vi "Find the boundary for Case Stucture.vi"(11 "Array 2":cluster{"Position":T1, "Bounds Rect":T2}[](array[cluster])) -> (0 "Height":i32, 1 "Width":i32, 2 "Top Min":i32, 3 "Left Min":i32)   [LabVIEW 2014]
uses:
  <vilib>/Utility/miscctls.llb/LVPositionTypeDef.ctl
  <vilib>/Utility/miscctls.llb/LVRectTypeDef.ctl
panel:
  out "Top Max":i32
  out "Left Max":i32
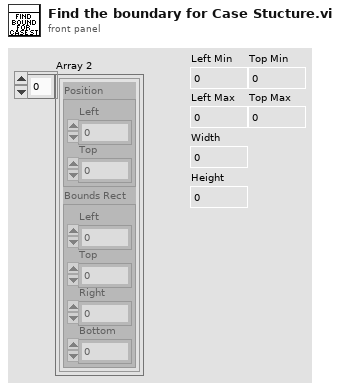
[diagram p1: front panel]
types:
  T1 = typedef "LVPositionTypeDef.ctl" = cluster{"Left":i32, "Top":i32}
  T2 = typedef "LVRectTypeDef.ctl" = cluster{"Left":i16, "Top":i16, "Right":i16, "Bottom":i16}
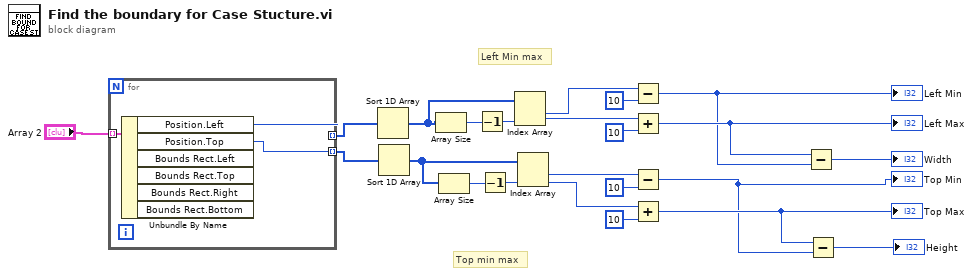
[diagram p0: block diagram]
diagram:
  # "Top min max"
  # "Left Min max"
  n1 = for {
    tunnel: "Array 2" -> [w26] mode=indexing
    tunnel: [w25] -> w23 mode=indexing
    tunnel: [w24] -> w22 mode=indexing
    n2 = Unbundle By Name(w26) -> ("Position.Left"=w25:i32, "Position.Top"=w24:i32)  [unwired: 4 out]
  }
  n3 = Sort 1D Array(array=w23) -> (sorted array=w20:i32[])
  n4 = Sort 1D Array(array=w22) -> (sorted array=w16:i32[])
  n5 = Array Size(array=w20) -> (size(s)=w21:i32)
  n6 = Array Size(array=w16) -> (size(s)=w17:i32)
  n7 = Decrement(x=w21) -> (x-1=w19:i32)
  n8 = Decrement(x=w17) -> (x-1=w18:i32)
  n9 = Index Array(array=w20, index #2=w19) -> (element #1=w15:i32, element #2=w9:i32)  [unwired: 1 in]
  n10 = Index Array(array=w16, index #2=w18) -> (element #1=w12:i32, element #2=w11:i32)  [unwired: 1 in]
  n11 = Subtract(x=w15, y=10 ("x")) -> (x-y=w4:i32)
  "Left Min" <- w4
  n12 = Add(x=w9, y=10 ("x")) -> (x+y=w7:i32)
  "Left Max" <- w7
  n13 = Subtract(x=w12, y=10 ("x")) -> (x-y=w2:i32)
  "Top Min" <- w2
  n14 = Add(x=w11, y=10 ("x")) -> (x+y=w6:i32)
  "Top Max" <- w6
  n15 = Subtract(x=w7, y=w4) -> (x-y=→"Width":i32)
  n16 = Subtract(x=w6, y=w2) -> (x-y=→"Height":i32)
